vi "Discovery Beacon Broadcast Loop.vi"(0 "name":string, 5 "TCP Server EndPoint":T1, 7 "discoveryPort":u16=10001, 9 "interval (ms)":u16=2000, 11 "kill thread notifier":refnum<notifier>) -> ()   [LabVIEW 2020, in "epl-network.lvlib"]
uses:
  epl-network.lvlib
  Public/TCP/Typedefs/IPEndPoint.ctl
  Public/Discovery/Typedefs/Server Beacon.ctl
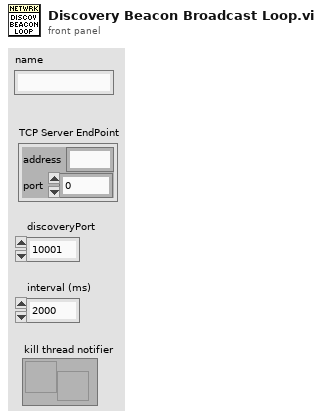
[diagram p1: front panel]
types:
  T1 = typedef "epl-network.lvlib/IPEndPoint.ctl" = cluster{"address":string, "port":i32}
  T2 = typedef "epl-network.lvlib/Server Beacon.ctl" = cluster{"name":string, "addr":string, "port":u16, "ver":u16}
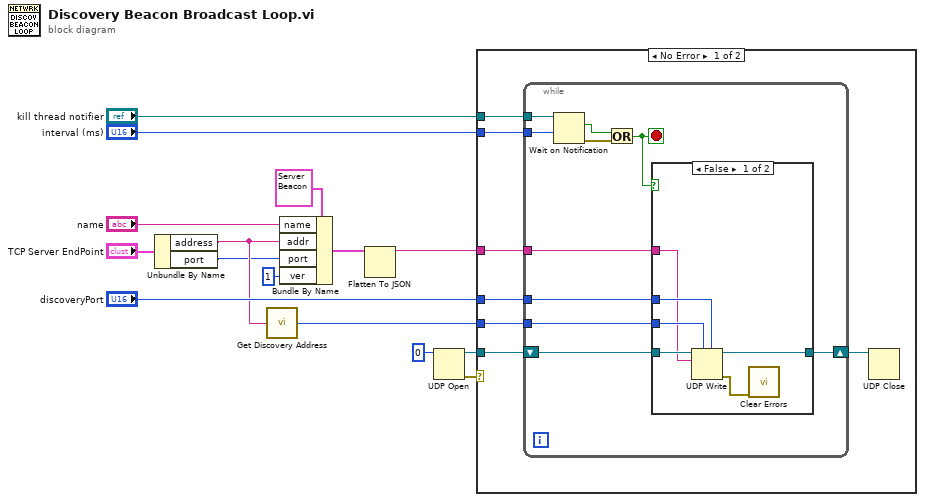
[diagram p0: block diagram]
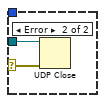
[diagram p3: hidden frame]
diagram:
  n1 = Unbundle By Name("TCP Server EndPoint") -> ("address"=w2:string, "port"=w1:i32)
  n2 = call "Get Discovery Address.vi"("Address"=w2) -> ("subnet address"=w7:u32)  [unwired: 13 in, 1 out]
  n3 = Bundle By Name(cluster=T2 {"name"="", "addr"="192.168.1.98", "port"=57469, "ver"=10001} ("DiscoveryBeacon"), "name"="name", "addr"=w2, "port"=w1, "ver"=u16 1 ("Version")) -> (w13:T2)
  n4 = Flatten To JSON(anything=w13) -> (JSON string=w6:string)  [unwired: 2 in, 1 out]
  n5 = UDP Open(11:0) -> (port=w9:refnum<k16>, 0:w8:errorcluster)  [unwired: 4 in, 1 out]
  n6 = case shown="No Error" w8 {
    selector: w8 -> [_ w41]
    tunnel: "kill thread notifier" -> [w22 _]
    tunnel: "interval (ms)" -> [w21 _]
    tunnel: w6 -> [w20 _]
    tunnel: w9 -> [w19 w40]
    tunnel: w7 -> [w18 _]
    tunnel: "discoveryPort" -> [w17 _]
    frame No Error {
      n7 = while {
        tunnel: w22 -> [w32]
        tunnel: w21 -> [w31]
        tunnel: w20 -> [w28]
        shift-right: [w24] -> w16
        shift-left: w19 -> [w27]
        tunnel: w18 -> [w26]
        tunnel: w17 -> [w25]
        stop <- w23 stop-if-true
        n8 = Wait on Notification(notifier=w32, timeout in ms (-1)=w31) -> (notification=w30:bool, error out=w29:errorcluster)  [unwired: 2 in, 2 out]
        n9 = Or(x=w30, y=w29) -> (x .or. y?=w23:bool)
        n10 = case shown="False" w23 {
          tunnel: w28 -> [w35 _]
          tunnel: w27 -> [w38 w39]
          tunnel: w26 -> [w37 _]
          tunnel: w25 -> [w36 _]
          tunnel: [w34 w39] -> w24
          frame False {
            n11 = UDP Write(address=w37, port or service name=w36, connection ID=w38, data in=w35) -> (error out=w33:errorcluster, 3:w34:refnum<k16>)  [unwired: 2 in]
            n12 = call <vilib>:"Clear Errors.vi"("error in (no error)"=w33) -> ()  [unwired: 5 in, 2 out]
          }
          frame True {
          }
        }
      }
      n13 = UDP Close(connection ID=w16) -> ()  [unwired: 1 in, 2 out]
    }
    frame Error {
      n14 = UDP Close(connection ID=w40, 8:w41) -> ()  [unwired: 2 out]
    }
  }
